vi "Create Spreadsheet of Event Names.vi"() -> ()   [LabVIEW 2013, in "FRCts20_SNS.lvlib"]
uses:
  FRCts20_SNS.lvlib
  FIRST Client/source/VI Source/FC_FIRST Client.lvlib
  FIRST Client/source/VI Source/FC_Target.ctl
  <vilib>/Utility/file.llb/Write To Spreadsheet File (string).vi
panel:
  out "Array":string[](array[string])
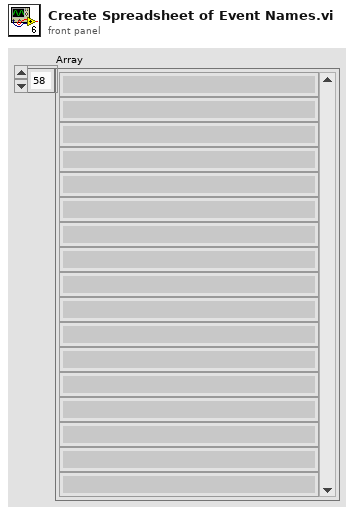
[diagram p1: front panel]
types:
  T1 = typedef "FC_FIRST Client.lvlib/FC_Target.ctl" = enum16{"Teams", "Competitions"}
  T2 = typedef "FC_FIRST Client.lvlib/FC_Competition Attributes.ctl" = cluster{"Event ID":string, "Event Name":string, "Venue":string, "City":string, "State":string, "Country":string, "Start Date":string, "End Date":string, "Year":string}
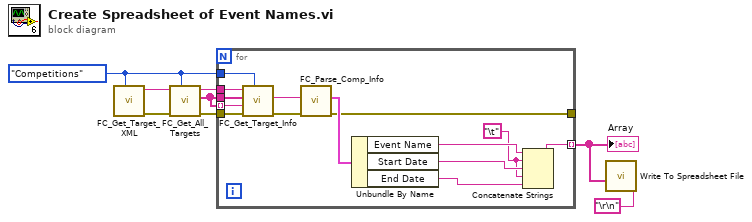
[diagram p0: block diagram]
diagram:
  w4 = FC_Target."Competitions" ("Target")
  n1 = call "FC_Get_Target_XML.vi"("Target"=w4) -> ("error out"=w7:errorcluster, "All Teams XML"=w8:string)  [unwired: 9 in]
  n2 = call "FC_Get_All_Targets.vi"("Target"=w4, "Error In"=w7, "Target XML"=w8) -> ("error out"=w5:errorcluster, "Array of Targets"=w6:string[], "Copy of Target XML"=w3:string)  [unwired: 6 in]
  n3 = for {
    tunnel: w6 -> [w22]
    tunnel: w6 -> [w21] mode=indexing
    tunnel: w5 -> [w20]
    tunnel: [w14] -> w2 mode=indexing
    tunnel: w4 -> [w16]
    tunnel: w3 -> [w15]
    tunnel: [w9] -> _
    w11 = "\t"
    n4 = call "FC_Get_Target_Info.vi"("Target"=w16, "Error In"=w20, "Desired Target"=w21, "Array of Targets"=w22, "Target XML"=w15) -> ("error out"=w19:errorcluster, "Target Info"=w18:string)  [unwired: 5 in]
    n5 = call "FC_Parse_Comp_Info.vi"("Error In"=w19, "All Competition Data"=w18) -> ("Error Out"=w9:errorcluster, "Comp Data Cluster"=w17:T2)  [unwired: 8 in]
    n6 = Unbundle By Name(w17) -> ("Event Name"=w13:string, "Start Date"=w12:string, "End Date"=w10:string)
    n7 = Concatenate Strings(w13, w11, w12, w11, w10) -> (w14:string)
  }
  "Array" <- w2
  n8 = call-poly <vilib>:"Write To Spreadsheet File.vi"("delimiter (\\t)"="\r\n", "1D data"=w2) -> ()  [unwired: 6 in, 1 out]
